vi "ColumnHeader.vi"(8 "error in":errorcluster, 9 "NomDon":string[](array[string])=["RTêta;", "X&Y;"], 10 "IndCourbe":i64 caption="Numéro de Balayage", 11 "Experiment.lvclass In":refnum<class "Experiment.lvclass">) -> (0 "error out":errorcluster, 2 "Scan list":string[](array[string]), 3 "Experiment.lvclass Out":refnum<class "Experiment.lvclass">, 4 "ScanTableSize":i32[](array[numeric]))   [LabVIEW 2010, in "Experiment.lvclass"]
doc: "Ce Vi créer la ligne d'entête du fichier texte de sauvegarde à partir du nombre de courbe voulu."
uses:
  Experiment.lvclass
  Experiment.lvclass/Experiment.ctl
  DevicesClass/BaseDevice/BaseDevice.lvclass
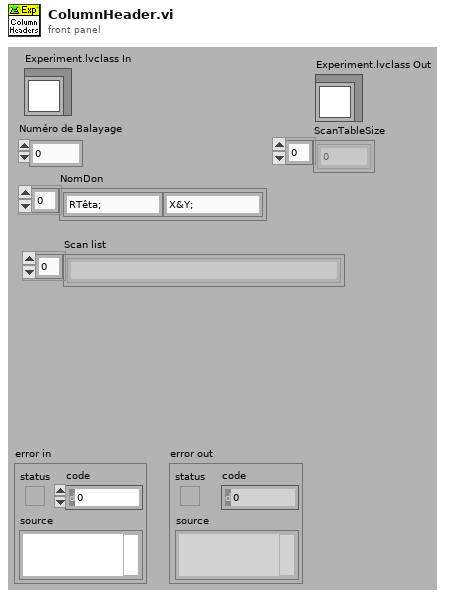
[diagram p1: front panel]
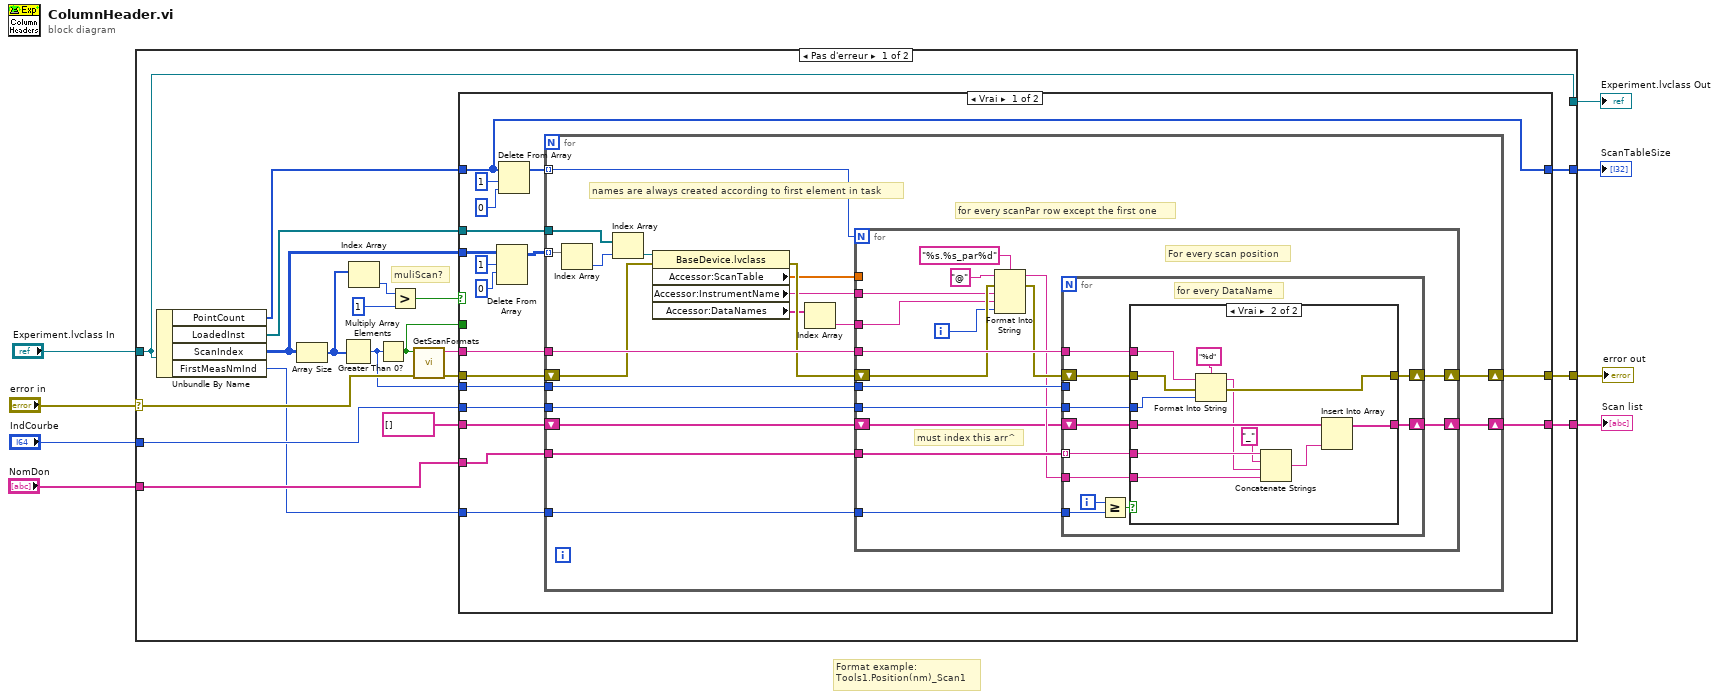
[diagram p0: block diagram]
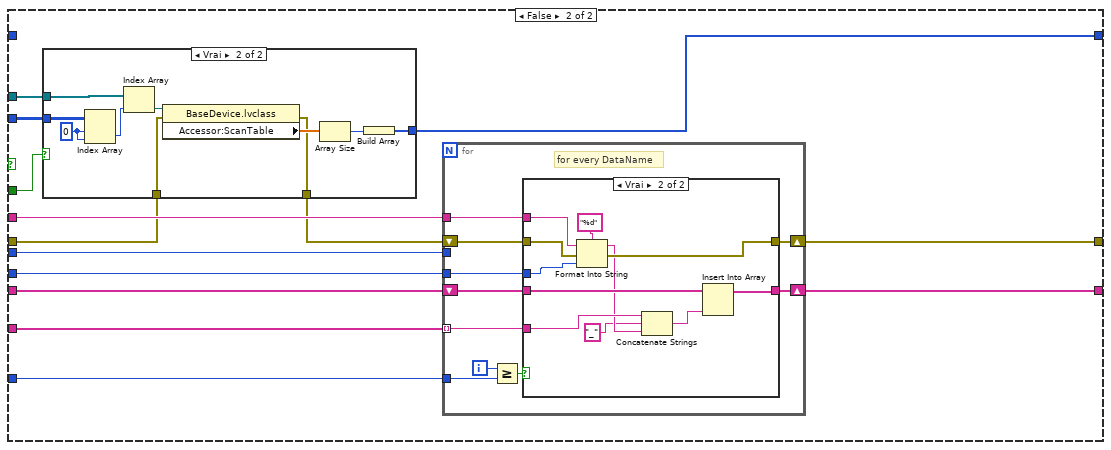
[diagram p3: hidden frame]
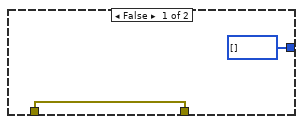
[diagram p4: hidden frame]
diagram:
  # "Format example:\nTools1.Position(nm)_Scan1"
  n1 = case shown="Pas d'erreur" "error in" {
    selector: "error in" -> [w28 w157]
    tunnel: [w17 w157] -> w7
    tunnel: [w23 _] -> w6
    tunnel: "NomDon" -> [w24 _]
    tunnel: "Experiment.lvclass In" -> [w14 w156]
    tunnel: "IndCourbe" -> [w26 _]
    tunnel: [w14 w156] -> w2
    tunnel: [w13 _] -> w1
    frame No Error {
      # "muliScan?"
      n2 = Unbundle By Name(w14) -> ("PointCount"=w9:i32[], "LoadedInst"=w18:refnum<class "BaseDevice.lvclass">[], "ScanIndex"=w19:i32[][], "FirstMeasNmInd"=w16:i32)
      n3 = Array Size(array=w19) -> (size(s)=w11:i32[])
      n4 = Multiply Array Elements(1:w11) -> (0:w21:i32)
      n5 = Index Array(array=w11) -> (element=w10:i32)  [unwired: 1 in]
      n6 = Greater Than 0?(x=w21) -> (x > 0?=w12:bool)
      n7 = Greater?(x=w10, y=1) -> (0:w15:bool)
      n8 = call "GetScanFormats.vi"("ErrorIn(No Error)"=w28, "Scan(T)"=w12) -> ("sortie d'erreur"=w25:errorcluster, "Prefixe"=w27:string)  [unwired: 7 in, 1 out]
      n9 = case shown="Vrai" w15 {
        tunnel: w27 -> [w46 w120]
        tunnel: w26 -> [w45 w119]
        tunnel: w25 -> [w44 w109]
        tunnel: w24 -> [w43 w118]
        tunnel: [w36 w117] -> w23
        tunnel: string[] [] -> [w37 w116]
        tunnel: w21 -> [w42 w115]
        tunnel: w19 -> [w41 w112]
        tunnel: w18 -> [w40 w111]
        tunnel: [w39 w114] -> w17
        tunnel: w16 -> [w38 w113]
        tunnel: [w29 w110] -> w13
        tunnel: w12 -> [_ w107]
        tunnel: w9 -> [w29 _]
        frame True {
          n10 = Delete From Array(array=w41, length=1 ("longueur"), index (row)=0 ("indice (ligne)")) -> (array with subset deleted=w35:i32[][])  [unwired: 1 in, 1 out]
          n11 = Delete From Array(array=w29, length=1 ("longueur"), index=0 ("indice")) -> (array with subset deleted=w32:i32[])  [unwired: 1 out]
          n12 = for {
            tunnel: w46 -> [w65]
            tunnel: w42 -> [w64]
            tunnel: w45 -> [w63]
            tunnel: w43 -> [w62]
            tunnel: w35 -> [w61] mode=indexing
            tunnel: w40 -> [w59]
            shift-right: [w55] -> w39
            shift-left: w44 -> [w57]
            tunnel: w38 -> [w54]
            shift-right: [w50] -> w36
            shift-left: w37 -> [w49]
            tunnel: w32 -> [w47] mode=indexing
            # "names are always created according to first element in task"
            # "for every scanPar row except the first one"
            n13 = Index Array(array=w61) -> (element=w60:i32)  [unwired: 1 in]
            n14 = Index Array(array=w59, index=w60) -> (element=w58:refnum<class "BaseDevice.lvclass">)
            n15 = property class="BaseDevice.lvclass"(reference=w58, error in=w57) -> (error out=w56:errorcluster, "Accessor:ScanTable"=w48:dbl[], "Accessor:InstrumentName"=w51:string, "Accessor:DataNames"=w53:string[])  [unwired: 1 out]
            n16 = Index Array(array=w53) -> (element=w52:string)  [unwired: 1 in]
            n17 = for {
              N: w47 -> [_]
              tunnel: w65 -> [w81]
              tunnel: w64 -> [w80]
              tunnel: w63 -> [w79]
              tunnel: w62 -> [w78]
              shift-right: [w76] -> w55
              shift-left: w56 -> [w73]
              tunnel: w54 -> [w75]
              tunnel: w52 -> [w71]
              tunnel: w51 -> [w70]
              shift-right: [w77] -> w50
              shift-left: w49 -> [w66]
              tunnel: w48 -> [_]
              i -> [w67]
              # "must index this arr^"
              # "For every scan position"
              n18 = Format Into String(format string="%s.%s_par%d" ("chaîne de format"), initial string="@" ("chaîne initiale"), error in=w73, w70, w71, w67) -> (resulting string=w68:string, error out=w72:errorcluster)
              n19 = for {
                tunnel: w81 -> [w87]
                tunnel: w78 -> [w90] mode=indexing
                shift-right: [w91] -> w77
                shift-left: w66 -> [w92]
                tunnel: w80 -> [_]
                tunnel: w79 -> [w88]
                shift-right: [w85] -> w76
                shift-left: w72 -> [w86]
                tunnel: w75 -> [w83]
                tunnel: w68 -> [w82]
                i -> [w84]
                # "for every DataName"
                n20 = Greater Or Equal?(x=w84, y=w83) -> (x >= y?=w89:bool)
                n21 = case shown="Vrai" w89 {
                  tunnel: w92 -> [w94 w106]
                  tunnel: [w94 w105] -> w91
                  tunnel: w90 -> [_ w104]
                  tunnel: w88 -> [_ w96]
                  tunnel: w87 -> [_ w103]
                  tunnel: w86 -> [w93 w102]
                  tunnel: [w93 w101] -> w85
                  tunnel: w82 -> [_ w97]
                  frame False {
                    # "in a scan the first items are the scanpar (var param): dont include it in graph legend"
                  }
                  frame True {
                    n22 = Format Into String(format string="%d" ("chaîne de format"), initial string=w103, error in=w102, w96) -> (resulting string=w99:string, error out=w101:errorcluster)
                    n23 = Concatenate Strings(w104, "_" ("chaîne"), w99, w97) -> (w100:string)
                    n24 = Insert Into Array(array=w106, new element=w100) -> (w105:string[])  [unwired: 1 in]
                  }
                }
              }
            }
          }
        }
        frame False {
          n25 = case shown="Vrai" w107 {
            tunnel: w112 -> [_ w130]
            tunnel: w111 -> [_ w128]
            tunnel: [i32[] [] w125] -> w110
            tunnel: w109 -> [w122 w124]
            tunnel: [w122 w123] -> w108
            frame False {
            }
            frame True {
              w129 = 0 ("indice (ligne)")
              n26 = Index Array(array=w130, index (row)=w129, index (col)=w129) -> (element=w132:i32)
              n27 = Index Array(array=w128, index=w132) -> (element=w131:refnum<class "BaseDevice.lvclass">)
              n28 = property class="BaseDevice.lvclass"(reference=w131, error in=w124) -> (error out=w123:errorcluster, "Accessor:ScanTable"=w127:dbl[])  [unwired: 1 out]
              n29 = Array Size(array=w127) -> (size(s)=w126:i32)
              n30 = Build Array(w126) -> (w125:i32[])
            }
          }
          n31 = for {
            tunnel: w120 -> [w137]
            tunnel: w118 -> [w140] mode=indexing
            shift-right: [w141] -> w117
            shift-left: w116 -> [w142]
            tunnel: w115 -> [_]
            tunnel: w119 -> [w138]
            shift-right: [w135] -> w114
            shift-left: w108 -> [w136]
            tunnel: w113 -> [w133]
            i -> [w134]
            # "for every DataName"
            n32 = Greater Or Equal?(x=w134, y=w133) -> (x >= y?=w139:bool)
            n33 = case shown="Vrai" w139 {
              tunnel: w142 -> [w144 w155]
              tunnel: [w144 w154] -> w141
              tunnel: w140 -> [_ w153]
              tunnel: w138 -> [_ w146]
              tunnel: w137 -> [_ w152]
              tunnel: w136 -> [w143 w151]
              tunnel: [w143 w150] -> w135
              frame False {
                # "in a scan the first items are the scanpar (var param): dont include it in graph legend"
              }
              frame True {
                n34 = Format Into String(format string="%d" ("chaîne de format"), initial string=w152, error in=w151, w146) -> (resulting string=w148:string, error out=w150:errorcluster)
                n35 = Concatenate Strings(w153, "_" ("chaîne"), w148) -> (w149:string)
                n36 = Insert Into Array(array=w155, new element=w149) -> (w154:string[])  [unwired: 1 in]
              }
            }
          }
        }
      }
    }
    frame Error {
    }
  }
  "error out" <- w7
  "Scan list" <- w6
  "Experiment.lvclass Out" <- w2
  "ScanTableSize" <- w1
